vi "EnumerateNumberOfDynamicModules.vi"(8 "error in (no error)":errorcluster, 11 "modules":T1[](array[typedef])) -> (0 "error out":errorcluster, 2 "number of dynamic modules":i32, 3 "all dynamic modules":string[](array[string]))   [LabVIEW 2017, in "CmsFpgaBitfileManager.lvlib"]
uses:
  <vilib>/addons/InsightCM/Devices/Shared/Cms/CmsFpgaBitfileManager/CmsFpgaBitfileManager.lvlib
  <vilib>/addons/cRIODetectHW/control/cRIO Product Info.ctl
  <vilib>/addons/cRIODetectHW/cRIODetectHW.lvlib
panel:
  out "all scan modules":string[](array[string])
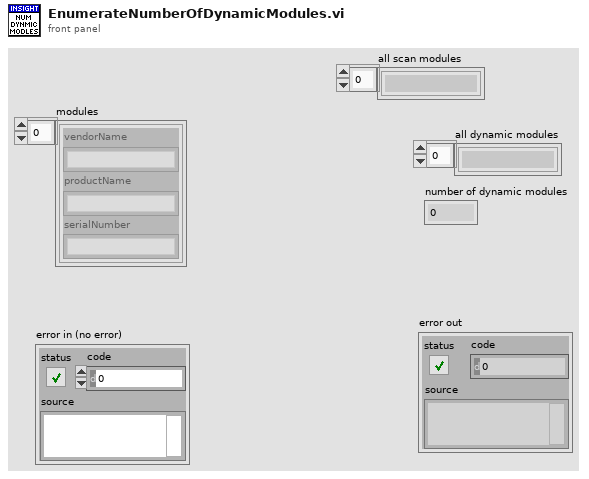
[diagram p1: front panel]
types:
  T1 = typedef "cRIODetectHW.lvlib/cRIO Product Info.ctl" = cluster{"vendorName":string, "productName":string, "serialNumber":string}
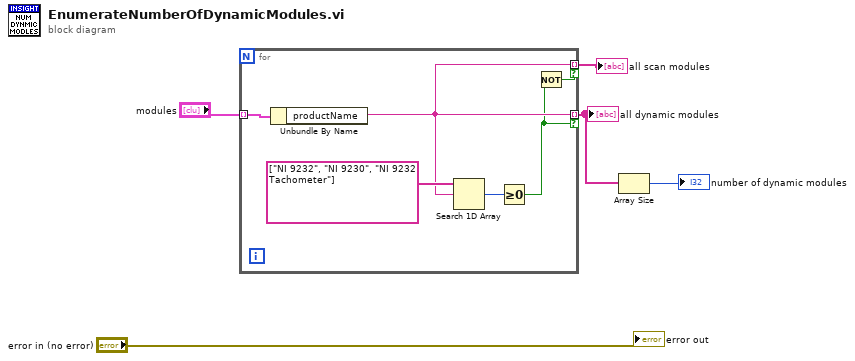
[diagram p0: block diagram]
diagram:
  n1 = for {
    tunnel: "modules" -> [w9] mode=indexing
    tunnel: [w8] -> w3 mode=indexing if=w7
    tunnel: [w8] -> w1 mode=indexing if=w6
    n2 = Unbundle By Name(w9) -> ("productName"=w8:string)
    n3 = Search 1D Array(1D array=string[] ["NI 9232", "NI 9230", "NI 9232 Tachometer"], element=w8) -> (index of element=w10:i32)  [unwired: 1 in]
    n4 = Greater Or Equal To 0?(x=w10) -> (x >= 0?=w7:bool)
    n5 = Not(x=w7) -> (.not. x?=w6:bool)
  }
  "all dynamic modules" <- w3
  "all scan modules" <- w1
  n6 = Array Size(array=w3) -> (size(s)=→"number of dynamic modules":i32)
  "error out" <- "error in (no error)"
